vi "Format MAC into String.vi"(11 "MAC":u8[](array[numeric])) -> (3 "MAC String":string)   [LabVIEW 2020, in "FrameEditor.lvlib"]
uses:
  FrameEditor.lvlib
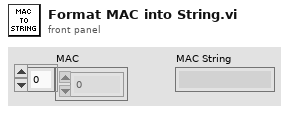
[diagram p1: front panel]
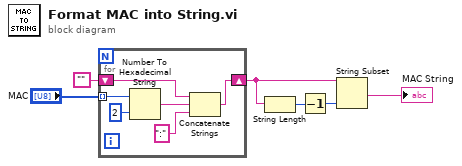
[diagram p0: block diagram]
diagram:
  n1 = for {
    tunnel: "MAC" -> [w12] mode=indexing
    shift-right: [w8] -> w6
    shift-left: "" -> [w7]
    n2 = Number To Hexadecimal String(1:i16 2 ("width (-)"), 2:w12) -> (0:w10:string)
    n3 = Concatenate Strings(w7, w10, ":" ("string")) -> (w8:string)
  }
  n4 = String Length(string=w6) -> (length=w4:i32)
  n5 = Decrement(x=w4) -> (x-1=w3:i32)
  n6 = String Subset(string=w6, length (rest)=w3) -> (substring=→"MAC String":string)  [unwired: 1 in]
